vi "ChangeSetup.vi"(8 "error in":errorcluster, 9 "Targets":T1 {"Select Mode:" items=["Custom", "Imaging", "300 All", "600 UV", "600 Blue", "600 Mid", "600 Red", "1200 m0", "1200 m1", "1200 m2", "1200 m3", "1200 m4", "1200 m5", "1200 m6", "1200 m7", "1200 RESOLVE", "400 m1", "400 m2", "930 m1", "930 m2", "930 m3", "930 m4", "930 m5", "930 m6", "400KL"]}, 11 "Script":T2[](array[typedef])) -> (0 "error out":errorcluster, 3 "Done":string)   [LabVIEW 2015]
uses:
  Script_actions.ctl
  Users/Sherman/Desktop/BETA_GSCS/Systems/Primary Filter/f1driveractions.ctl
  Users/Sherman/Desktop/BETA_GSCS/Systems/Secondary Filter/f2driveractions.ctl
  Users/Sherman/Desktop/BETA_GSCS/Systems/Coll_Focus/coll_actions.ctl
  Users/Sherman/Desktop/BETA_GSCS/Systems/Wavelength/wavelength_parameters.ctl
  Users/Sherman/Desktop/BETA_GSCS/Systems/Wavelength/movetypes.ctl
  Users/Sherman/Desktop/BETA_GSCS/Systems/Wavelength/wavelength_driver_actions.ctl
  Users/Sherman/Desktop/BETA_GSCS/Systems/Grating_Translation/GTdriveractions.ctl
  Users/Sherman/Desktop/BETA_GSCS/Systems/Slit/slitactions.ctl
  Users/Sherman/Desktop/BETA_GSCS/Systems/Cam_Focus/CF_drivercontrol.ctl
  Utils/GSP_Wavelength_Global.vi
  Users/Sherman/Desktop/BETA_GSCS/Systems/Primary Filter/GSP_F1_Global.vi
  Users/Sherman/Desktop/BETA_GSCS/Systems/Secondary Filter/GSP_F2_Global.vi
  Users/Sherman/Desktop/BETA_GSCS/Systems/Coll_Focus/GSP_COLL_Global.vi
  Users/Sherman/Desktop/BETA_GSCS/Systems/Grating_Translation/GSP_GT_Global.vi
  Users/Sherman/Desktop/BETA_GSCS/Systems/Slit/GSP_SLIT_Global.vi
  Users/Sherman/Desktop/BETA_GSCS/Systems/Cam_Focus/GSP_CF_Global.vi
panel:
  out "VI Refnum":refnum<vi>
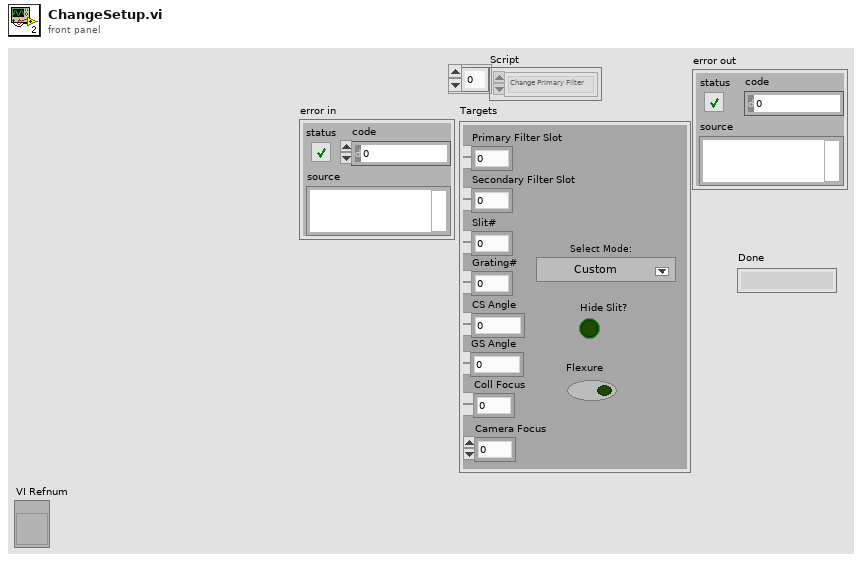
[diagram p1: front panel]
types:
  T1 = cluster{"Primary Filter Slot":i32, "Secondary Filter Slot":i32, "Slit#":i32, "Grating#":i32, "CS Angle":dbl, "GS Angle":dbl, "Coll Focus":i32, "Camera Focus":i32, "Select Mode:":u16, "Flexure":bool, "Hide Slit?":bool}
  T2 = typedef "Script_actions.ctl" = enum16{"Change Primary Filter", "Change Secondary Filter", "Change Collimator Focus", "Change Camera Focus", "Change Grating", "Change Angles", "Change Slit Mask", "Toggle Slit", "Change WAVMODE", "Check All Systems", "Change Flexure"}
  T3 = typedef "f1driveractions.ctl" = enum16{"Launch", "INIT_CTL", "Home", "Move", "Shutdown"}
  T4 = typedef "f2driveractions.ctl" = enum16{"Launch", "INIT_CTL", "Home", "Move", "Shutdown"}
  T5 = typedef "coll_actions.ctl" = enum16{"Launch", "Move", "Home", "Open Shutter", "Close Shutter", "Shutdown"}
  T6 = typedef "wavelength_driver_actions.ctl" = enum16{"Launch", "Flexure On", "Flexure Off", "Move", "Home", "Shutdown"}
  T7 = typedef "wavelength_parameters.ctl" = cluster{"Camera Angle":dbl, "Grating  Angle":dbl, "Move type":T8}
  T8 = typedef "movetypes.ctl" = u16
  T9 = typedef "GTdriveractions.ctl" = enum16{"Launch", "INIT_CTL", "Move", "Home", "Shutdown"}
  T10 = typedef "slitactions.ctl" = enum16{"Launch", "INIT_CTL", "Restart", "Show", "Hide", "Home", "Move", "Rotate Only", "Shutdown"}
  T11 = typedef "CF_drivercontrol.ctl" = enum16{"Launch", "Move", "Set Piezos", "Flexure On", "Flexure Off", "Home", "Shutdown"}
  T12 = typedef "ThreadStates.ctl" = enum16{"Waiting", "Scripting", "Uninitialized", "Error"}
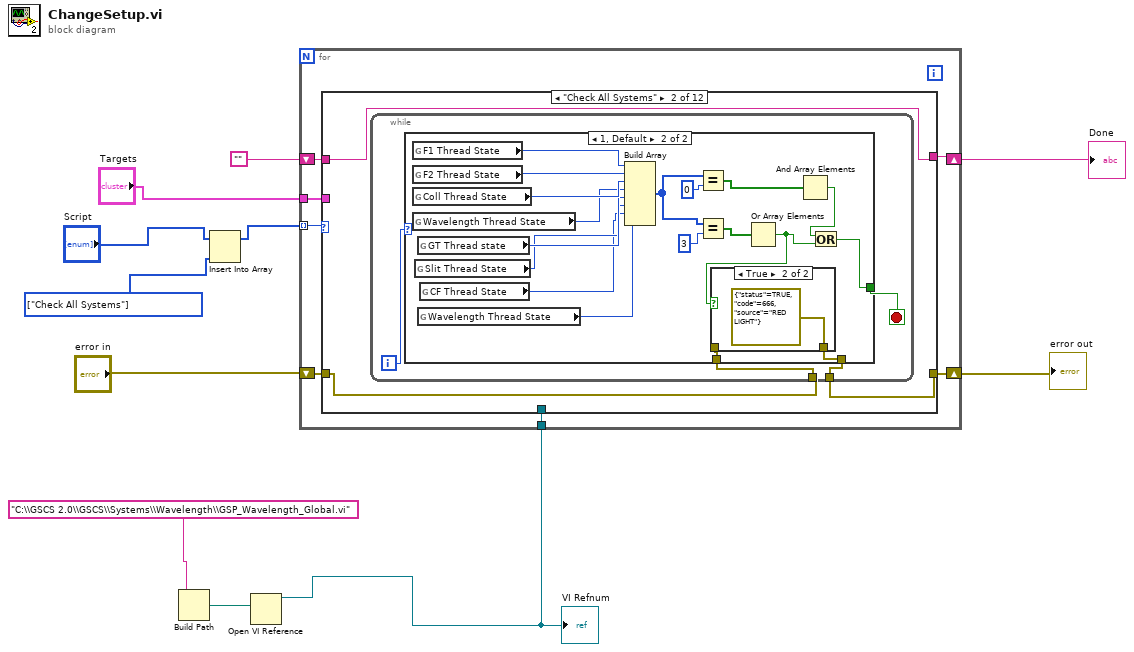
[diagram p0: block diagram]
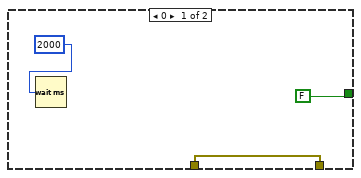
[diagram p3: hidden frame]
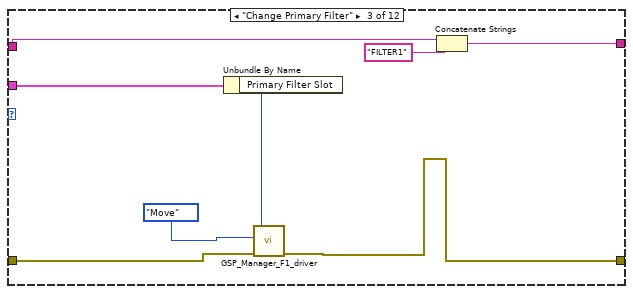
[diagram p5: hidden frame]
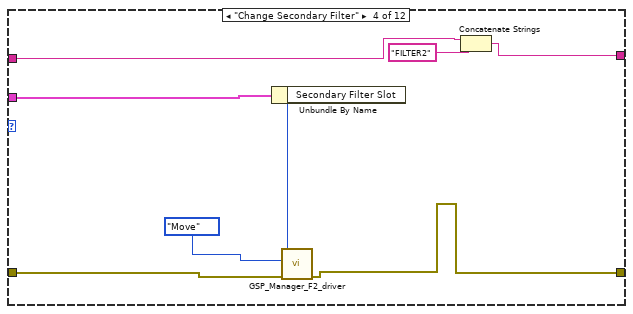
[diagram p6: hidden frame]
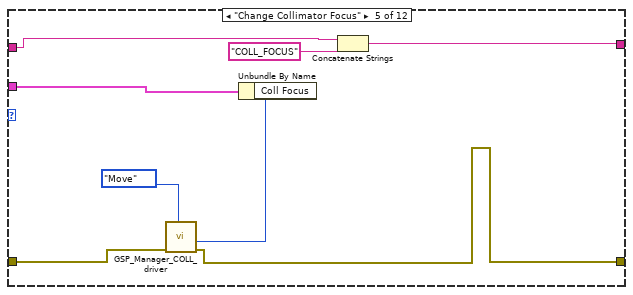
[diagram p7: hidden frame]
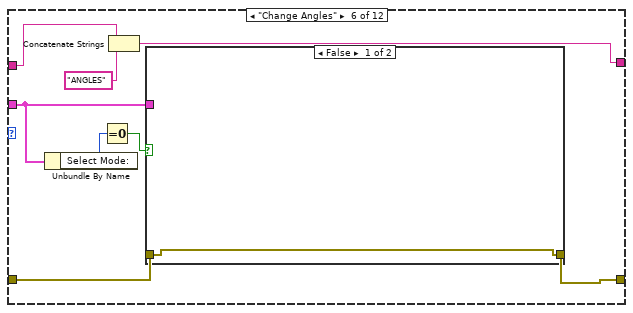
[diagram p8: hidden frame]
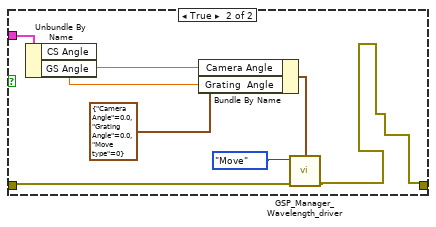
[diagram p9: hidden frame]
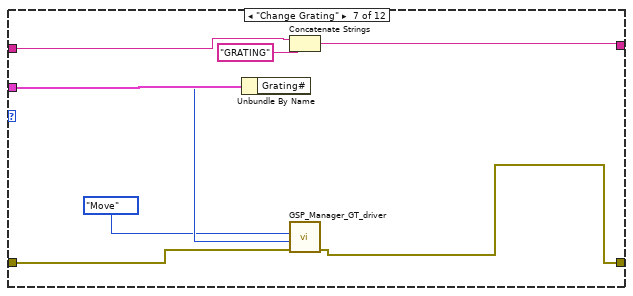
[diagram p10: hidden frame]
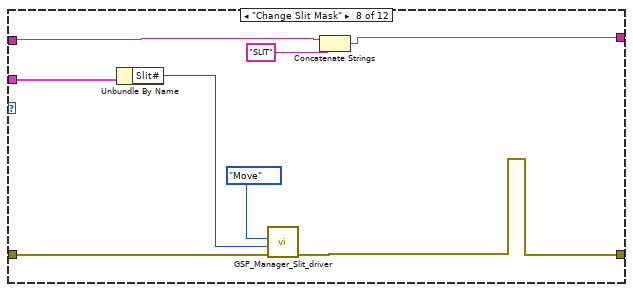
[diagram p11: hidden frame]
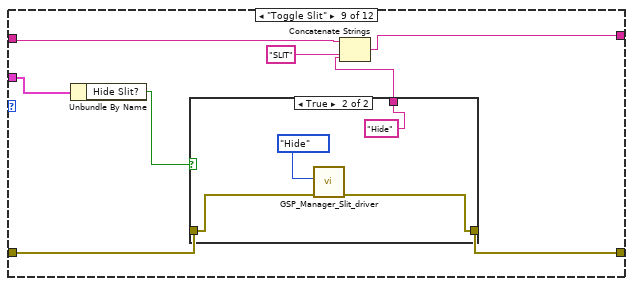
[diagram p12: hidden frame]
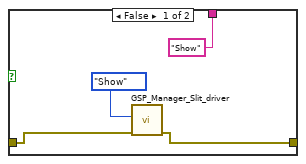
[diagram p13: hidden frame]
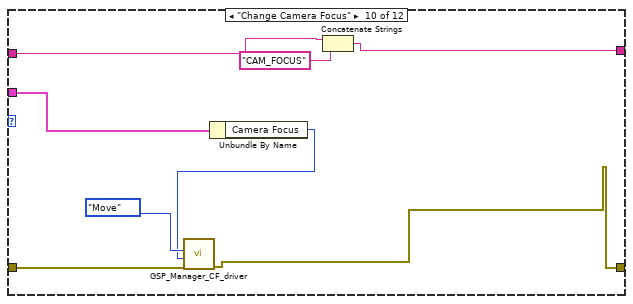
[diagram p14: hidden frame]
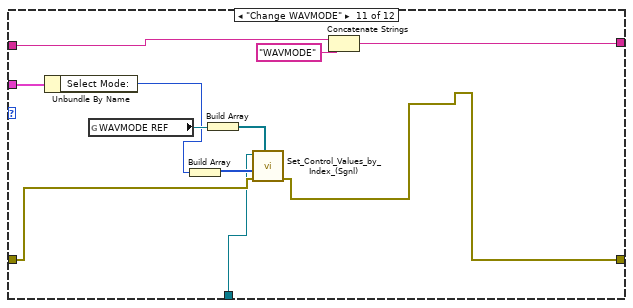
[diagram p15: hidden frame]
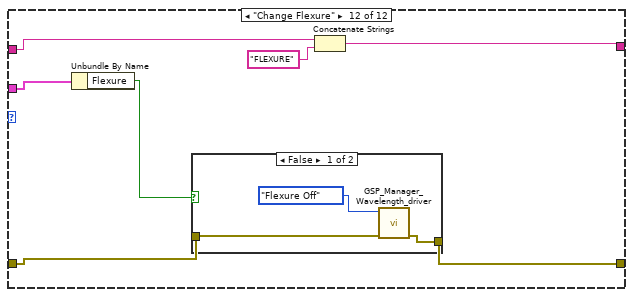
[diagram p16: hidden frame]
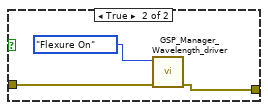
[diagram p17: hidden frame]
diagram:
  w4 = T2[] [enum."Check All Systems"] items=["Change Primary Filter", "Change Secondary Filter", "Change Collimator Focus", "Change Camera Focus", "Change Grating", "Change Angles", "Change Slit Mask", "Toggle Slit", "Change WAVMODE", "Check All Systems", "Change Flexure"]
  n1 = Build Path(name or relative path="C:\\GSCS 2.0\\GSCS\\Systems\\Wavelength\\GSP_Wavelength_Global.vi" ("vi path")) -> (appended path=w8:path)  [unwired: 1 in]
  n2 = Insert Into Array(array="Script", new element=w4) -> (w5:T2[])  [unwired: 1 in]
  n3 = Open VI Reference(vi path=w8) -> (vi reference=w1:refnum<vi>)  [unwired: 5 in, 1 out]
  "VI Refnum" <- w1
  n4 = for {
    tunnel: w5 -> [w17] mode=indexing
    shift-right: [w15] -> w9
    shift-left: "error in" -> [w18]
    tunnel: "Targets" -> [w16]
    shift-right: [w13] -> w2
    shift-left: "" -> [w14]
    tunnel: w1 -> [w12]
    n5 = case shown="\"Check All Systems\"" w17 {
      tunnel: w18 -> [w20 w23 w57 w65 w73 w82 w98 w106 w111 w131 w137 w149]
      tunnel: w16 -> [_ _ w58 w66 w74 w80 w99 w107 w112 w130 w142 w147]
      tunnel: [w20 w22 w54 w62 w70 w81 w95 w103 w110 w127 w136 w148] -> w15
      tunnel: w14 -> [w19 w21 w53 w60 w68 w76 w93 w101 w114 w125 w134 w145]
      tunnel: [w19 w21 w52 w59 w67 w75 w92 w100 w113 w124 w133 w143] -> w13
      tunnel: w12 -> [_ _ _ _ _ _ _ _ _ _ w132 _]
      frame Default {
      }
      frame "Check All Systems" {
        n6 = while {
          tunnel: w23 -> [w25]
          tunnel: [w24] -> w22
          i -> [w26]
          stop <- w27 stop-if-true
          n7 = case shown="1, Default" w26 {
            tunnel: [FALSE w34] -> w27
            tunnel: w25 -> [w28 w33]
            tunnel: [w28 w32] -> w24
            frame 0 {
              n8 = Wait (ms)(milliseconds to wait=2000) -> ()  [unwired: 1 out]
            }
            frame 1, Default {
              n9 = global read "GSP_F1_Global.vi" "F1 Thread State"() -> (w48:T12)
              n10 = global read "GSP_F2_Global.vi" "F2 Thread State"() -> (w47:T12)
              n11 = global read "GSP_COLL_Global.vi" "Coll Thread State"() -> (w46:T12)
              n12 = global read "GSP_Wavelength_Global.vi" "Wavelength Thread State"() -> (w45:T12)
              n13 = global read "GSP_SLIT_Global.vi" "Slit Thread State"() -> (w43:T12)
              n14 = global read "GSP_GT_Global.vi" "GT Thread state"() -> (w44:T12)
              n15 = global read "GSP_Wavelength_Global.vi" "Wavelength Thread State"() -> (w41:T12)
              n16 = global read "GSP_CF_Global.vi" "CF Thread State"() -> (w42:T12)
              n17 = Build Array(w48, w47, w46, w45, w44, w43, w42, w41) -> (w40:T12[])
              n18 = Equal?(x=w40, y=0) -> (x = y?=w37:bool[])
              n19 = Equal?(x=w40, y=3) -> (x = y?=w36:bool[])
              n20 = Or Array Elements(Boolean array=w36) -> (logical OR=w31:bool)
              n21 = case shown="True" w31 {
                tunnel: w33 -> [w49 _]
                tunnel: [w49 errorcluster {"status"=TRUE, "code"=666, "source"="RED LIGHT"} ("error constant")] -> w32
                frame False {
                }
                frame True {
                }
              }
              n22 = And Array Elements(Boolean array=w37) -> (logical AND=w35:bool)
              n23 = Or(x=w35, y=w31) -> (x .or. y?=w34:bool)
            }
          }
        }
      }
      frame "Change Primary Filter" {
        n24 = Unbundle By Name(w58) -> ("Primary Filter Slot"=w56:i32)
        n25 = call "GSP_Manager_F1_driver.vi"("error in (no error)"=w57, "Action"=f1driveractions."Move", "Filter# (Move Only)"=w56) -> ("error out"=w54:errorcluster)  [unwired: 3 in, 1 out]
        n26 = Concatenate Strings(w53, "FILTER1") -> (w52:string)
      }
      frame "Change Secondary Filter" {
        n27 = Unbundle By Name(w66) -> ("Secondary Filter Slot"=w63:i32)
        n28 = call "GSP_Manager_F2_driver.vi"("error in (no error)"=w65, "Action"=f2driveractions."Move", "Filter# (Move Only)"=w63) -> ("error out"=w62:errorcluster)  [unwired: 3 in, 1 out]
        n29 = Concatenate Strings(w60, "FILTER2") -> (w59:string)
      }
      frame "Change Collimator Focus" {
        n30 = Unbundle By Name(w74) -> ("Coll Focus"=w72:i32)
        n31 = call "GSP_Manager_COLL_driver.vi"("error in (no error)"=w73, "Target (Move Only)"=w72, "Action"=coll_actions."Move") -> ("error out"=w70:errorcluster)  [unwired: 3 in, 1 out]
        n32 = Concatenate Strings(w68, "COLL_FOCUS") -> (w67:string)
      }
      frame "Change Angles" {
        n33 = Unbundle By Name(w80) -> ("Select Mode:"=w78:u16)
        n34 = Equal To 0?(x=w78) -> (x = 0?=w79:bool)
        n35 = Concatenate Strings(w76, "ANGLES") -> (w75:string)
        n36 = case shown="False" w79 {
          tunnel: w82 -> [w83 w91]
          tunnel: w80 -> [_ w88]
          tunnel: [w83 w84] -> w81
          frame False {
          }
          frame True {
            n37 = Unbundle By Name(w88) -> ("CS Angle"=w87:dbl, "GS Angle"=w86:dbl)
            n38 = Bundle By Name(cluster=T7 {"Camera Angle"=0.0, "Grating  Angle"=0.0, "Move type"=0} ("Target (Move Only)"), "Camera Angle"=w87, "Grating  Angle"=w86) -> (w89:T7)
            n39 = call "GSP_Manager_Wavelength_driver.vi"("error in (no error)"=w91, "Target (Move Only)"=w89, "Action"=wavelength_driver_actions."Move") -> ("error out"=w84:errorcluster)  [unwired: 3 in, 1 out]
          }
        }
      }
      frame "Change Grating" {
        n40 = Unbundle By Name(w99) -> ("Grating#"=w97:i32)
        n41 = Concatenate Strings(w93, "GRATING") -> (w92:string)
        n42 = call "GSP_Manager_GT_driver.vi"("error in (no error)"=w98, "Grating # (Move Only)"=w97, "Action"=GTdriveractions."Move") -> ("error out"=w95:errorcluster)  [unwired: 3 in, 1 out]
      }
      frame "Change Slit Mask" {
        n43 = Unbundle By Name(w107) -> ("Slit#"=w105:i32)
        n44 = call "GSP_Manager_Slit_driver.vi"("error in (no error)"=w106, "Slit # (Move/Rotate Only)"=w105, "Action"=slitactions."Move") -> ("error out"=w103:errorcluster)  [unwired: 3 in, 1 out]
        n45 = Concatenate Strings(w101, "SLIT") -> (w100:string)
      }
      frame "Toggle Slit" {
        n46 = Unbundle By Name(w112) -> ("Hide Slit?"=w109:bool)
        n47 = case shown="True" w109 {
          tunnel: w111 -> [w118 w122]
          tunnel: [w117 w121] -> w110
          tunnel: ["Show" "Hide"] -> w108
          frame False {
            n48 = call "GSP_Manager_Slit_driver.vi"("error in (no error)"=w118, "Action"=slitactions."Show") -> ("error out"=w117:errorcluster)  [unwired: 4 in, 1 out]
          }
          frame True {
            n49 = call "GSP_Manager_Slit_driver.vi"("error in (no error)"=w122, "Action"=slitactions."Hide") -> ("error out"=w121:errorcluster)  [unwired: 4 in, 1 out]
          }
        }
        n50 = Concatenate Strings(w114, "SLIT", w108) -> (w113:string)
      }
      frame "Change Camera Focus" {
        n51 = Unbundle By Name(w130) -> ("Camera Focus"=w128:i32)
        n52 = call "GSP_Manager_CF_driver.vi"("error in (no error)"=w131, "Target (Move Only)"=w128, "Action"=CF_drivercontrol."Move") -> ("error out"=w127:errorcluster)  [unwired: 4 in, 1 out]
        n53 = Concatenate Strings(w125, "CAM_FOCUS") -> (w124:string)
      }
      frame "Change WAVMODE" {
        n54 = Unbundle By Name(w142) -> ("Select Mode:"=w138:u16)
        n55 = global read "GSP_Wavelength_Global.vi" "WAVMODE REF"() -> (w141:refnum<vi>)
        n56 = Build Array(w138) -> (w139:u16[])
        n57 = Build Array(w141) -> (w140:refnum<vi>[])
        n58 = call "Set_Control_Values_by_Index_(Sgnl).vi"("Control References"=w140, "error in (no error)"=w137, "appended array"=w139, "VI Refnum"=w132) -> ("error out"=w136:errorcluster)  [unwired: 6 in, 1 out]
        n59 = Concatenate Strings(w134, "WAVMODE") -> (w133:string)
      }
      frame "Change Flexure" {
        n60 = Unbundle By Name(w147) -> ("Flexure"=w146:bool)
        n61 = case shown="False" w146 {
          tunnel: w149 -> [w151 w154]
          tunnel: [w150 w153] -> w148
          frame False {
            n62 = call "GSP_Manager_Wavelength_driver.vi"("error in (no error)"=w151, "Action"=wavelength_driver_actions."Flexure Off") -> ("error out"=w150:errorcluster)  [unwired: 4 in, 1 out]
          }
          frame True {
            n63 = call "GSP_Manager_Wavelength_driver.vi"("error in (no error)"=w154, "Action"=wavelength_driver_actions."Flexure On") -> ("error out"=w153:errorcluster)  [unwired: 4 in, 1 out]
          }
        }
        n64 = Concatenate Strings(w145, "FLEXURE") -> (w143:string)
      }
    }
  }
  "error out" <- w9
  "Done" <- w2
